vi "Array_2D_Reduce_Sum_Dim=1(CuLab).vi"(8 "error in (no error)":errorcluster, 11 "x":refnum<class "T2D_SGL.lvclass">) -> (0 "error out":errorcluster, 3 "y out":refnum<class "T1D_SGL.lvclass">)   [LabVIEW 2020]
uses:
  <vilib>/Ngene/CuLab - GPU Accelerated Toolkit/Toolkit/Low_Level/Tensor_Classes/T_Children/T1D/T1D_Children/T1D_SGL/T1D_SGL.lvclass
  C:/Program Files/National Instruments/LabVIEW 2020/vi.lib/Ngene/CuLab - GPU Accelerated Toolkit/Toolkit/Low_Level/Tensor_Classes/T_Children/T1D/T1D.lvclass
  <vilib>/Ngene/CuLab - GPU Accelerated Toolkit/Toolkit/Low_Level/Tensor_Classes/T_Children/T2D/T2D_Children/T2D_SGL/T2D_SGL.lvclass
  C:/Program Files/National Instruments/LabVIEW 2020/vi.lib/Ngene/CuLab - GPU Accelerated Toolkit/Toolkit/Low_Level/Tensor_Classes/T_Children/T2D/T2D.lvclass
  <vilib>/Ngene/CuLab - GPU Accelerated Toolkit/Toolkit/Low_Level/GPU_Wrapper/cublas/Controls/cublasOperation_t.ctl
  <vilib>/Ngene/CuLab - GPU Accelerated Toolkit/Toolkit/API/Array/Array Size/CU_Array_Size_T2D.vi
  <vilib>/Ngene/CuLab - GPU Accelerated Toolkit/Toolkit/API/Linear Algebra/BLAS2/gemv/CU_gemv/CU_Sgemv.vi
  <vilib>/Ngene/CuLab - GPU Accelerated Toolkit/Toolkit/CuLab.lvlib
  <vilib>/Ngene/Deep Learning Toolkit/Toolkit/Deep_Learning_Toolkit_by_Ngene.lvlib
  C:/Program Files/National Instruments/LabVIEW 2020/vi.lib/Ngene/CuLab - GPU Accelerated Toolkit/Toolkit/Low_Level/Tensor_Classes/Tensor.lvclass
  C:/Program Files/National Instruments/LabVIEW 2020/vi.lib/Ngene/CuLab - GPU Accelerated Toolkit/Toolkit/Low_Level/Tensor_Classes/T_Children/T2D/T2D_Children/T2D_SGL/T2D_SGL.lvclass
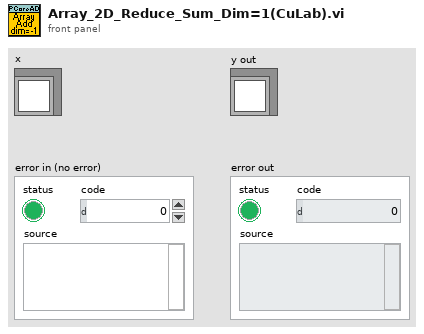
[diagram p1: front panel]
types:
  T1 = typedef "CuLab.lvlib/cublasOperation_t.ctl" = enum16{"Direct", "Transposed", "Conjugated & Transposed"}
  T2 = typedef "CuLab.lvlib/T2D_Dims.ctl" = cluster{"H":i32, "W":i32}
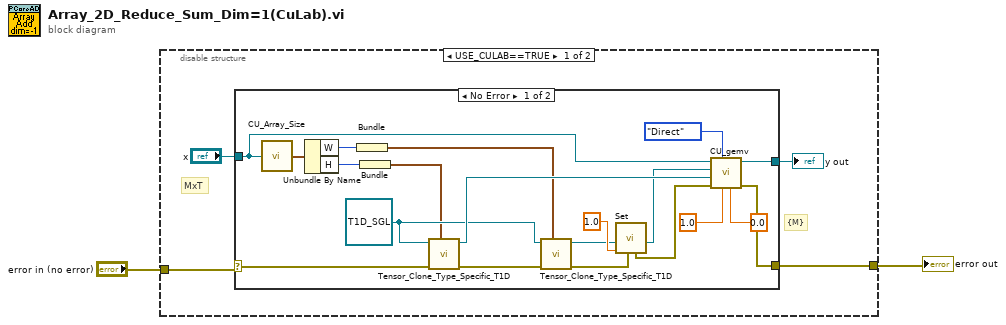
[diagram p0: block diagram]
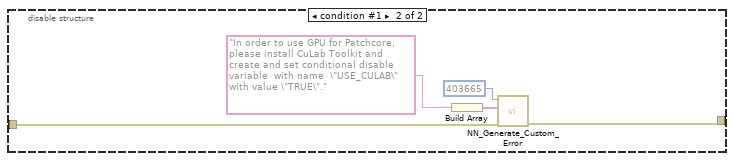
[diagram p3: hidden frame]
diagram:
  n1 = disable-structure shown="USE_CULAB==TRUE" {
    disable-tunnel: "error in (no error)" -> [w4 w29]
    disable-tunnel: [w3 w28] -> w1
    frame condition #0 (active) {
      # "{M}"
      # "MxT"
      n2 = case shown="No Error" w4 {
        selector: w4 -> [w24 w27]
        tunnel: "x" -> [w26 _]
        tunnel: [w25 _] -> w5
        tunnel: [w8 w27] -> w3
        frame No Error {
          w16 = refnum<class "T1D_SGL.lvclass"> refnum ("y")
          n3 = call-poly <vilib>:"CU_Array_Size.vi"("Tensor"=w26) -> ("T2D_Dims"=w21:T2)  [unwired: 14 in]
          n4 = Unbundle By Name(w21) -> ("W"=w9:i32, "H"=w20:i32)
          n5 = Bundle("W"=w9) -> (w10:cluster{"W":i32})  [unwired: 1 in]
          n6 = Bundle("H"=w20) -> (w13:cluster{"H":i32})  [unwired: 1 in]
          n7 = call <vilib>:"Tensor_Clone_Type_Specific_T1D.vi"("Dest_Tensor_Dims"=w13, "error in (no error)"=w24, "Dest_Tensor"=w16) -> ("error out"=w12:errorcluster, "Dest_Tensor out"=w18:refnum<class "T1D_SGL.lvclass">)  [unwired: 7 in]
          n8 = call <vilib>:"Tensor_Clone_Type_Specific_T1D.vi"("Dest_Tensor_Dims"=w10, "error in (no error)"=w12, "Dest_Tensor"=w16) -> ("error out"=w15:errorcluster, "Dest_Tensor out"=w17:refnum<class "T1D_SGL.lvclass">)  [unwired: 7 in]
          n9 = call <vilib>:"Set.vi"("error in (no error)"=w15, "Value"=sgl 1.0, "T1D_SGL in"=w17) -> ("T1D_SGL out"=w7:refnum<class "T1D_SGL.lvclass">, "error out"=w14:errorcluster)  [unwired: 7 in]
          n10 = call-poly <vilib>:"CU_gemv.vi"("beta"=sgl 0.0, "alpha"=sgl 1.0, "operation A"=cublasOperation_t."Direct", "error in (no error)"=w14, "y"=w18, "x"=w7, "A"=w26) -> ("error out"=w8:errorcluster, "y out"=w25:refnum<class "T1D_SGL.lvclass">)  [unwired: 3 in]
        }
        frame Error {
        }
      }
      "y out" <- w5
    }
    frame condition #1 {
      n11 = Build Array("In order to use GPU for Patchcore, please install CuLab Toolkit and create and set conditional disable variable  with name  \"USE_CULAB\" with value \"TRUE\"." ("Message")) -> (w31:string[])
      n12 = call <vilib>:"NN_Generate_Custom_Error.vi"("error in (no error)"=w29, "Message"=w31, "Error_code"=403665) -> ("error out"=w28:errorcluster)  [unwired: 8 in]
    }
  }
  "error out" <- w1
